vi "set-bscale.vi"(10 "bscale":dbl=1.0 min=0.0001 max=1.0 step=0.0001 format="%#_13g") -> (0 "error out":errorcluster)   [LabVIEW 2014]
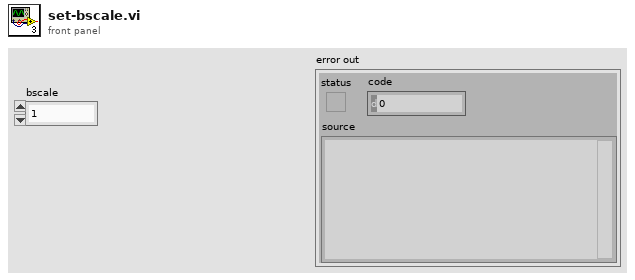
[diagram p1: front panel]
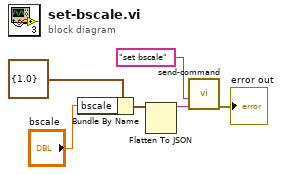
[diagram p0: block diagram]
diagram:
  n1 = Bundle By Name(cluster=cluster{"bscale":dbl} {"bscale"=1.0}, "bscale"="bscale") -> (w1:cluster{"bscale":dbl})
  n2 = Flatten To JSON(anything=w1) -> (JSON string=w5:string)  [unwired: 2 in, 1 out]
  n3 = call "send-command.vi"("parameters"=w5, "command"="set bscale") -> ("error out"=→"error out":errorcluster)  [unwired: 8 in, 1 out]
